vi "dimensions.vi"() -> ()   [LabVIEW 2015, in "Index JSON Array.xnode"]
uses:
  Index JSON Array.xnode
panel:
  in  "header.h":i16=19
  in  "footer.h":i16=8
  in  "element.h":i16=8
  in  "resize.v":i32=8
  in  "min.h":i32=35
  in  "min.w":i32=32
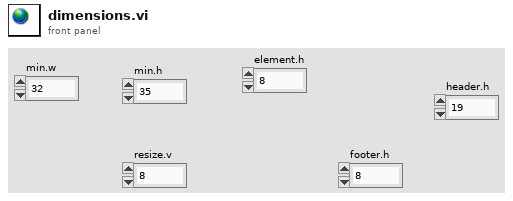
[diagram p1: front panel]
diagram:
